vi "1_3_real exponential sequence.vi"(1 "alpha":dbl=0.5, 2 "c":dbl=1.0, 3 "n":i32=40) -> (0 "?":dbl[](graph)=[1.0, 0.5, 0.25, 0.125, 0.0625, 0.03125, 0.015625, 0.0078125, 0.00390625, 0.001953125, 0.0009765625, 0.00048828125, 0.000244140625, 0.0001220703125, 6.103515625e-05, 3.0517578125e-05, 1.52587890625e-05, 7.62939453125e-06, 3.814697265625e-06, 1.9073486328125e-06, 9.5367431640625e-07, 4.76837158203125e-07, 2.384185791015625e-07, 1.1920928955078125e-07, 5.960464477539063e-08, 2.9802322387695312e-08, 1.4901161193847656e-08, 7.450580596923828e-09, 3.725290298461914e-09, 1.862645149230957e-09, 9.313225746154785e-10, 4.656612873077393e-10, 2.3283064365386963e-10, 1.1641532182693481e-10, 5.820766091346741e-11, 2.9103830456733704e-11, 1.4551915228366852e-11, 7.275957614183426e-12, 3.637978807091713e-12, 1.8189894035458565e-12])   [LabVIEW 2009]
doc: "This VI creates an array of n sample sequence given by the equation\nx[n] = C*alpha^n."
panel:
  in  "stop":bool
  # "Program Developed by Indranil Sinharoy"
  # "x[n] = c*alpha^n"
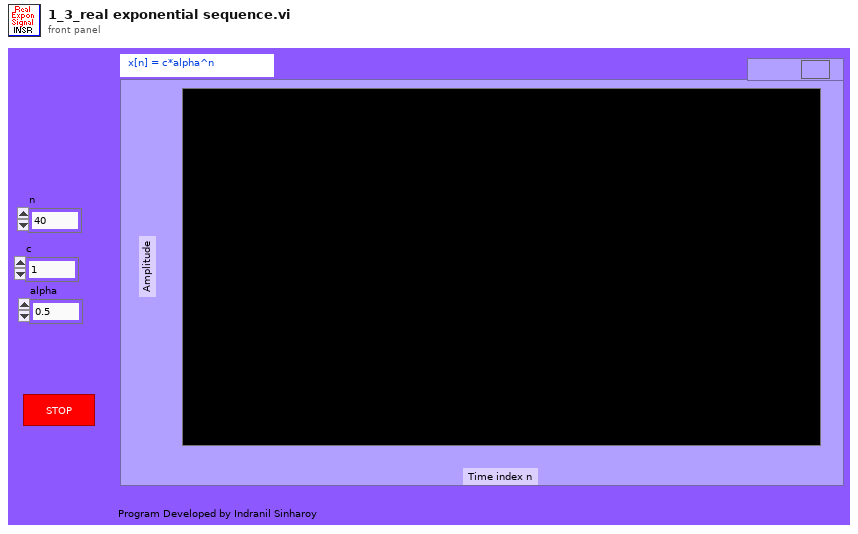
[diagram p1: front panel]
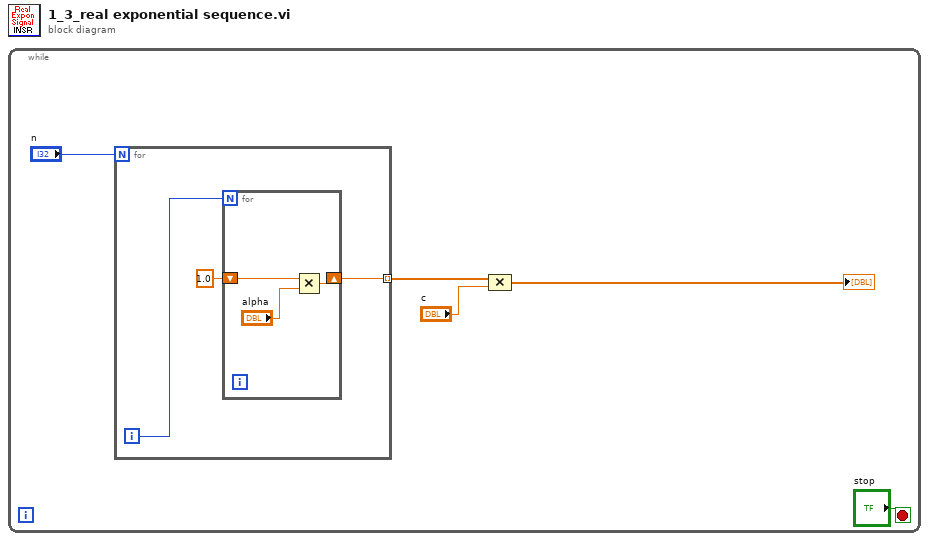
[diagram p0: block diagram]
diagram:
  n1 = while {
    stop <- "stop" stop-if-true
    n2 = for {
      N: "n" -> [_]
      tunnel: [w6] -> w4 mode=indexing
      i -> [w7]
      n3 = for {
        N: w7 -> [_]
        shift-right: [w10] -> w6
        shift-left: 1.0 -> [w9]
        n4 = Multiply(x=w9, y="alpha") -> (x*y=w10:dbl)
      }
    }
    n5 = Compound Arithmetic op=MULTIPLY(w4, "c") -> (→"?":dbl[])
  }
